vi "odczyt_danych_z_MCU.vi"(11 "VISA Refnum in":refnum<visa-resource-name>) -> (1 "read buffer 2":string, 2 "Boolean":bool, 3 "VISA Refnum out":refnum<visa-resource-name>, 4 "Boolean 2":bool, 5 "read buffer":string, 6 "read buffer 3":string)   [LabVIEW 2025]
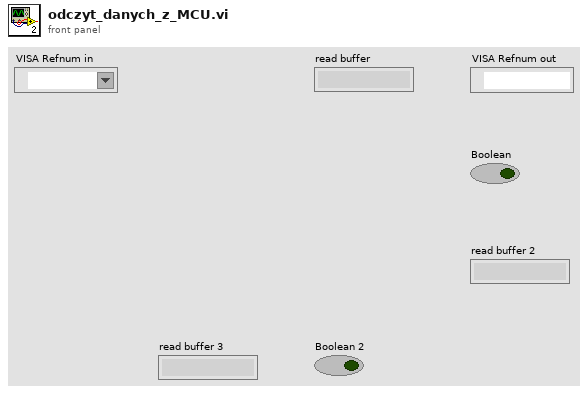
[diagram p1: front panel]
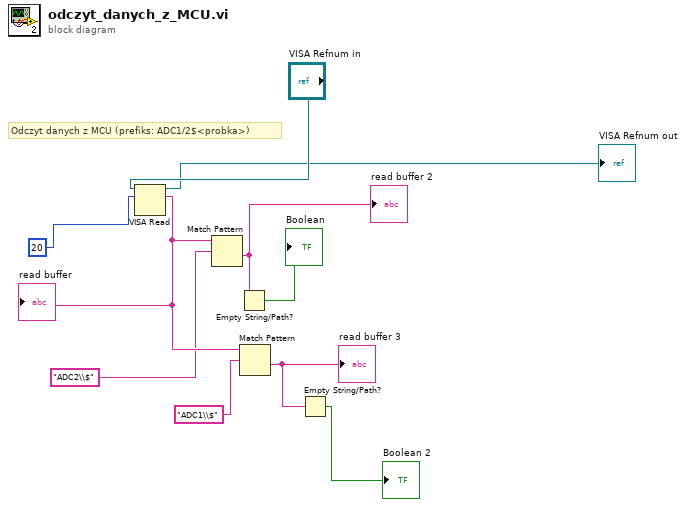
[diagram p0: block diagram]
diagram:
  # "Odczyt danych z MCU (prefiks: ADC1/2$<probka>)"
  n1 = VISA Read(VISA resource name="VISA Refnum in", byte count=u32 20) -> (VISA resource name out=→"VISA Refnum out":refnum<visa-resource-name>, read buffer=w9:string)  [unwired: 1 in, 2 out]
  "read buffer" <- w9
  n2 = Match Pattern(string=w9, regular expression="ADC2\\$") -> (after substring=w7:string)  [unwired: 1 in, 3 out]
  "read buffer 2" <- w7
  n3 = Empty String/Path?(string/path=w7) -> (empty?=→"Boolean":bool)
  n4 = Match Pattern(string=w9, regular expression="ADC1\\$") -> (after substring=w6:string)  [unwired: 1 in, 3 out]
  "read buffer 3" <- w6
  n5 = Empty String/Path?(string/path=w6) -> (empty?=→"Boolean 2":bool)
